vi "GV_AutoScale.vi"(8 "error in (no error)":errorcluster, 9 "AutoScale":T1, 11 "Gviewer in":refnum<class "Gviewer.lvclass">) -> (0 "error out":errorcluster, 3 "Gviewer out":refnum<class "Gviewer.lvclass">)   [LabVIEW 2020, in "Sgraph_lib_V1.lvlib" / "Gviewer.lvclass"]
doc: "Andre Koelewijn, 16 aug 2021\nPerform Autoscale action\nFix 29 dec 2021: skip autoscale if no data is present."
uses:
  Gviewer.lvclass
  controls/AutoScale.ctl
  Gviewer.lvclass/Gviewer.ctl
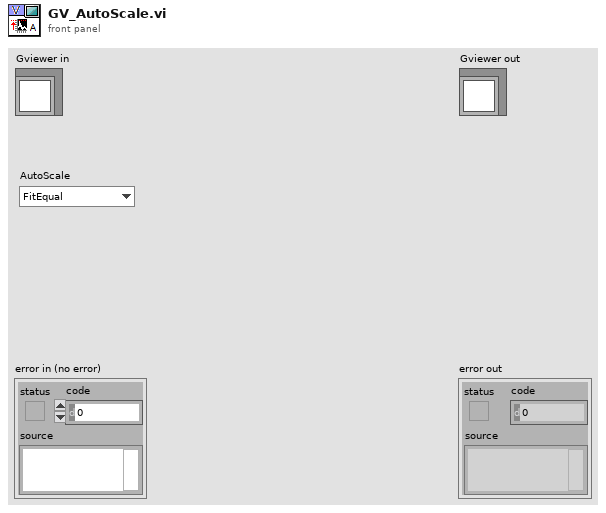
[diagram p1: front panel]
types:
  T1 = typedef "Sgraph_lib_V1.lvlib/Gviewer.lvclass/AutoScale.ctl" = enum16{"FitEqual", "FitMax", "StackEqual", "StackMax", "StackPerType"}
  T2 = typedef "Sgraph_lib_V1.lvlib/DBAL.lvclass/DBAL_TAGprops.ctl" = T3[]
  T3 = typedef "Sgraph_lib_V1.lvlib/DBAL.lvclass/DBAL_TAGpropEdit.ctl" = cluster{"TAG":string, "Qtype":string, "TAGprop":T4}
  T4 = typedef "Sgraph_lib_V1.lvlib/typedef_com_TagProp.ctl" = cluster{"Description":string, "EngUnits":string, "RangeH":dbl, "RangeL":dbl, "Resolution":i32, "Obsolete":bool, "ChangeDate":timestamp, "ChangeSource":string, "ChangeReason":string, "TagFunc":u32}
  T5 = cluster{"data":dbl[], "max":dbl[], "min":dbl[], "Status":u32[]}[]
  T6 = cluster{"data":dbl[], "max":dbl[], "min":dbl[], "Status":u32[]}
  T7 = typedef "Sgraph_lib_V1.lvlib/Gviewer.lvclass/Typedef_SelProperties.ctl" = cluster{"Color":u32, "LineType":T8, "max":dbl, "min":dbl}
  T8 = typedef "Sgraph_lib_V1.lvlib/Gviewer.lvclass/Typedef_LineType.ctl" = enum16{"num_bare", "num_MinMax_Area", "num_MinMax_Lines", "num_MinMax_Forfor", "num_Max_Area", "num_Max_Line", "num_Max_Forfor", "num_Min_Area", "num_Min_Line", "num_Min_Fosfor", "Boolean_Line_01", "Boolean_Area_01", "Boolean_Fosfor_01", "Boolean_Line_TF", "Boolean_Area_TF", "Boolean_Fosfor_TF", "Boolean_OnOff_Line", "Boolean_OnOff_Area", "Boolean_OnOff_Fosfor", "Boolean_spare", "StringEvent_Line", "StringEvent_TimeLine"}
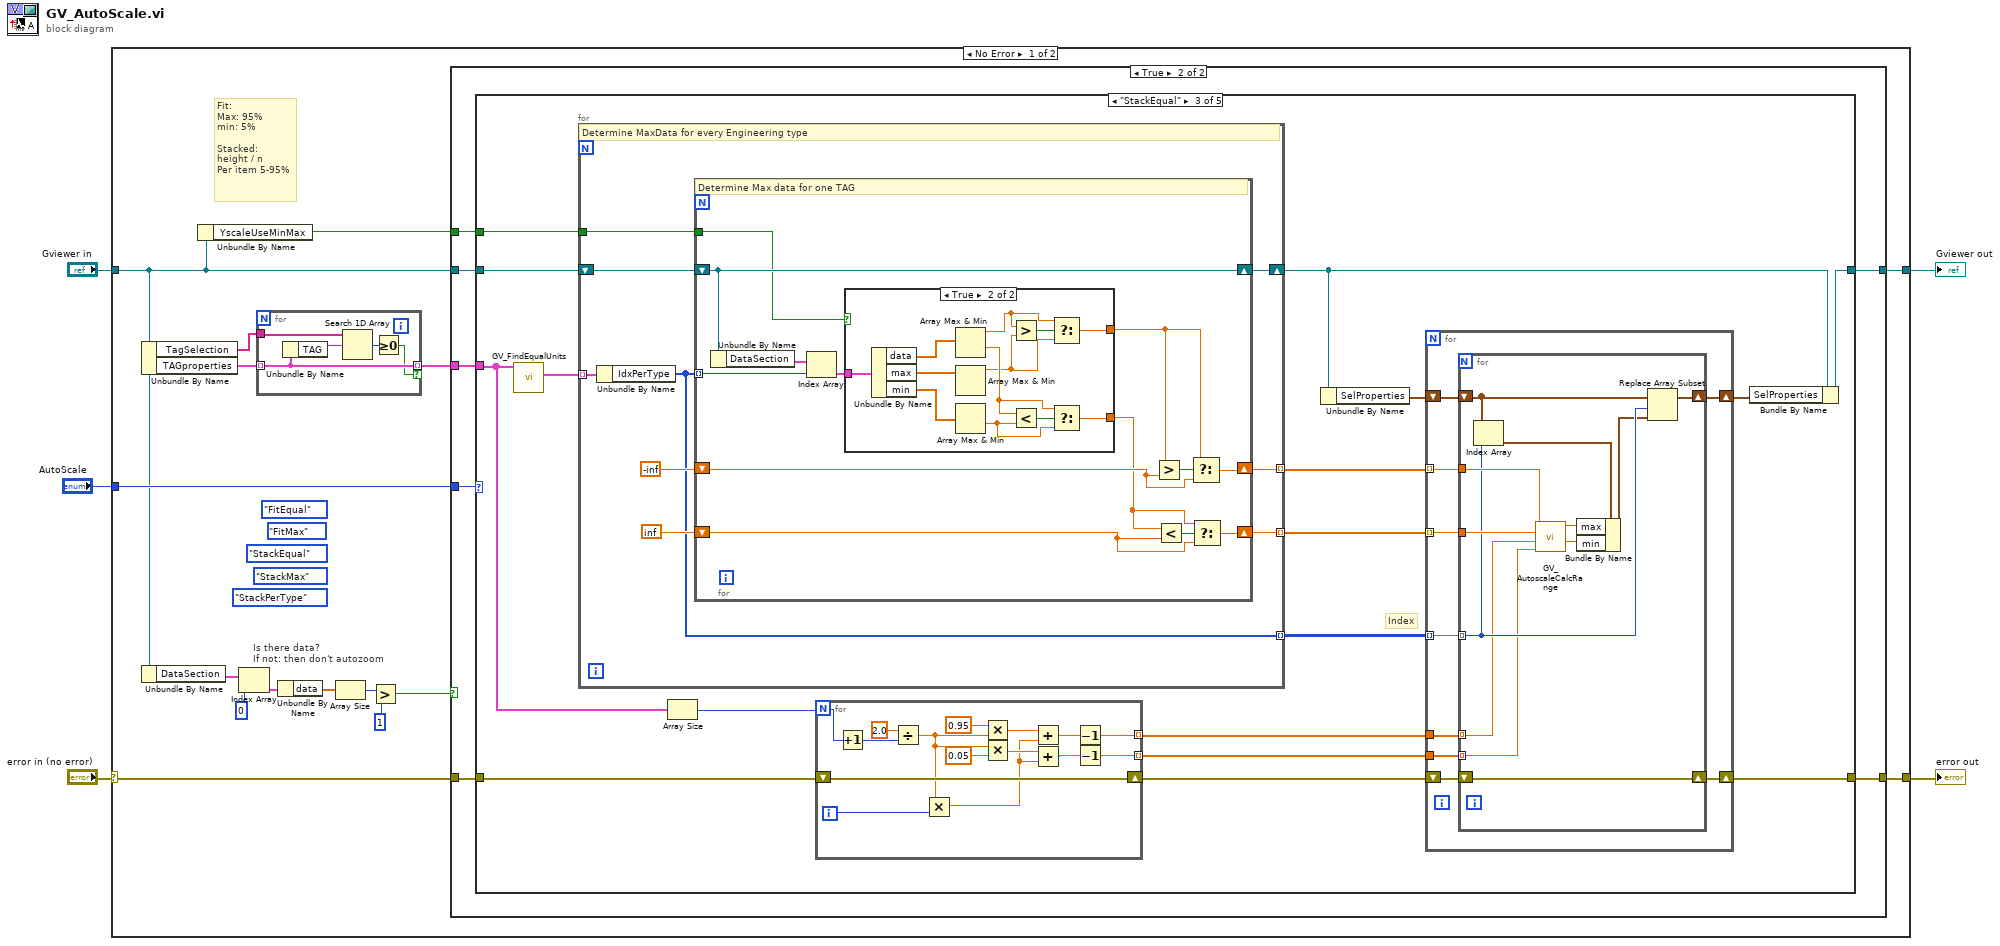
[diagram p0: block diagram]
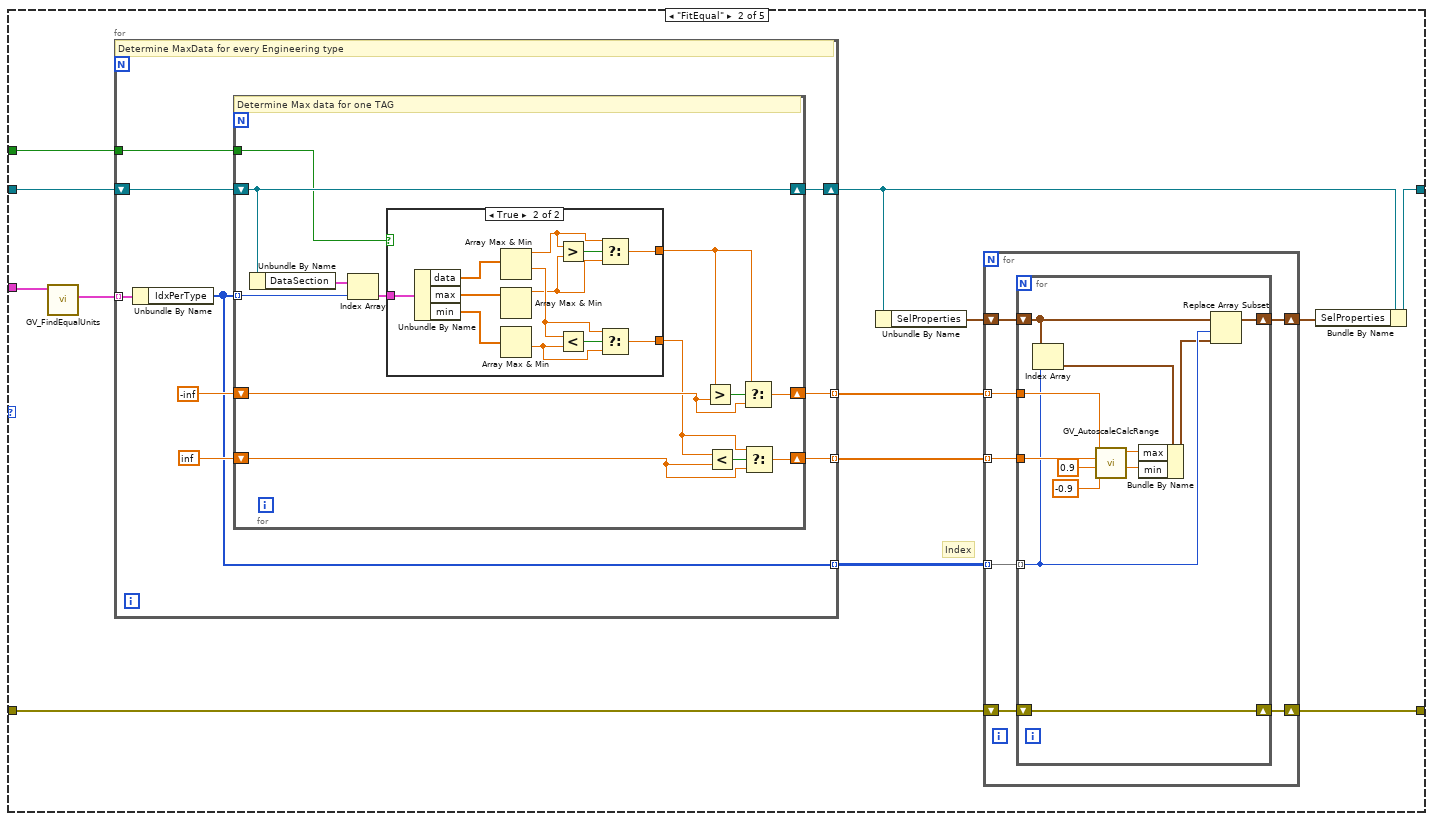
[diagram p4: hidden frame]
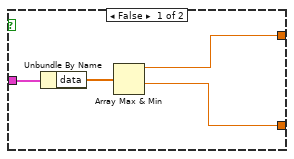
[diagram p5: hidden frame]
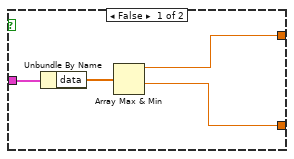
[diagram p6: hidden frame]
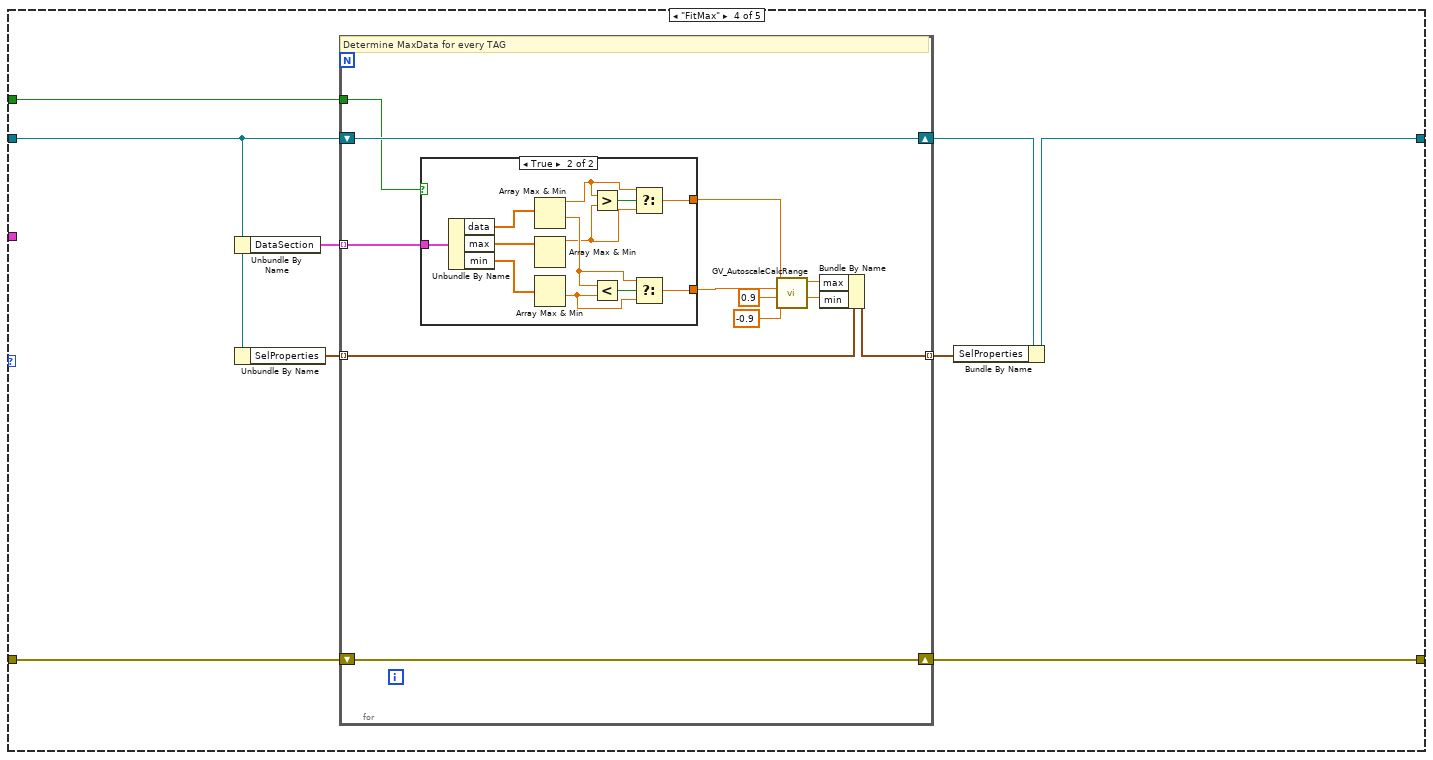
[diagram p7: hidden frame]
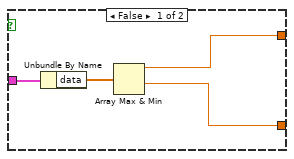
[diagram p8: hidden frame]
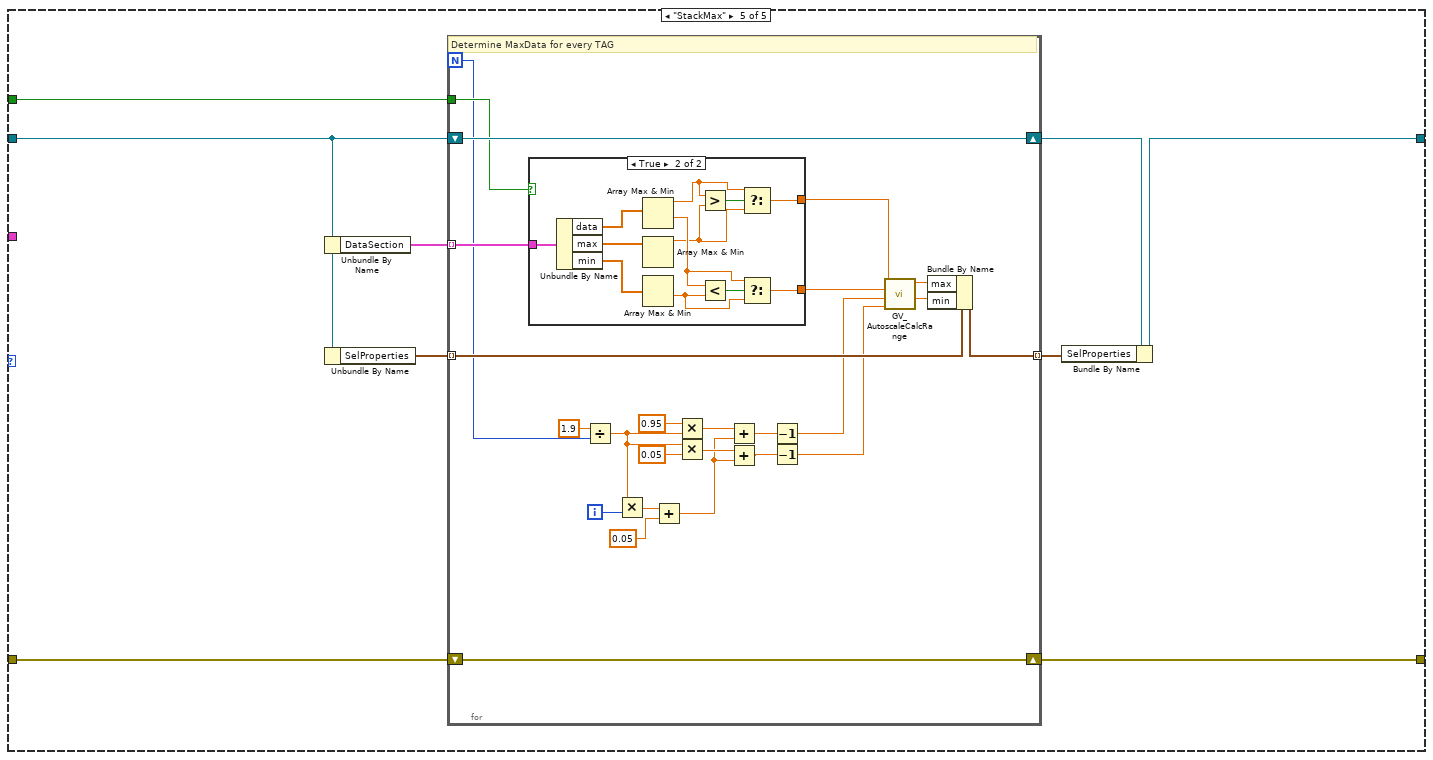
[diagram p9: hidden frame]
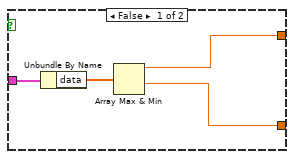
[diagram p10: hidden frame]
diagram:
  n1 = case shown="No Error" "error in (no error)" {
    selector: "error in (no error)" -> [w15 w284]
    tunnel: [w19 w284] -> w4
    tunnel: [w16 w283] -> w2
    tunnel: "Gviewer in" -> [w13 w283]
    tunnel: "AutoScale" -> [w17 _]
    frame No Error {
      (unwired) AutoScale."StackPerType" ("AutoScale")
      (unwired) AutoScale."StackMax" ("AutoScale")
      (unwired) AutoScale."StackEqual" ("AutoScale")
      (unwired) AutoScale."FitMax" ("AutoScale")
      (unwired) AutoScale."FitEqual" ("AutoScale")
      # "Is there data?\nIf not: then don't autozoom"
      # "Fit:\nMax: 95%\nmin: 5%\n\nStacked:\nheight / n\nPer item 5-95%"
      n2 = Unbundle By Name(w13) -> ("TagSelection"=w20:string[], "TAGproperties"=w21:T2)
      n3 = Unbundle By Name(w13) -> ("DataSection"=w12:T5)
      n4 = Unbundle By Name(w13) -> ("YscaleUseMinMax"=w14:bool)
      n5 = Index Array(array=w12, index=0) -> (element=w10:T6)
      n6 = for {
        tunnel: w21 -> [w282] mode=indexing
        tunnel: [w282] -> w18 mode=indexing if=w278
        tunnel: w20 -> [w281]
        n7 = Unbundle By Name(w282) -> ("TAG"=w280:string)
        n8 = Search 1D Array(1D array=w281, element=w280) -> (index of element=w279:i32)  [unwired: 1 in]
        n9 = Greater Or Equal To 0?(x=w279) -> (x >= 0?=w278:bool)
      }
      n10 = Unbundle By Name(w10) -> ("data"=w9:dbl[])
      n11 = Array Size(array=w9) -> (size(s)=w8:i32)
      n12 = Greater?(x=w8, y=1) -> (0:w6:bool)
      n13 = case shown="True" w6 {
        tunnel: [w22 w30] -> w19
        tunnel: w18 -> [_ w29]
        tunnel: w17 -> [_ w28]
        tunnel: [w23 w27] -> w16
        tunnel: w15 -> [w22 w26]
        tunnel: w14 -> [_ w25]
        tunnel: w13 -> [w23 w24]
        frame False {
        }
        frame True {
          n14 = case shown="\"StackEqual\"" w28 {
            tunnel: w26 -> [w32 w39 w104 w195 w234]
            tunnel: [w32 w39 w104 w191 w230] -> w30
            tunnel: w29 -> [_ w44 w106 _ _]
            tunnel: w24 -> [w31 w42 w115 w197 w228]
            tunnel: [w31 w33 w107 w192 w231] -> w27
            tunnel: w25 -> [_ w41 w114 w199 w236]
            frame Default {
            }
            frame "FitEqual" {
              # "Index"
              n15 = call "GV_FindEqualUnits.vi"("TAGproperties"=w44) -> ("IndexPerType"=w43:cluster{"EngUnit":string, "IdxPerType":i32[]}[])  [unwired: 8 in, 2 out]
              n16 = for {
                tunnel: w43 -> [w72] mode=indexing
                shift-right: [w71] -> w34
                shift-left: w42 -> [w70]
                tunnel: [w67] -> w38 mode=indexing
                tunnel: [w66] -> w37 mode=indexing
                tunnel: [w65] -> w40 mode=indexing
                tunnel: w41 -> [w64]
                # "Determine MaxData for every Engineering type"
                n17 = Unbundle By Name(w72) -> ("IdxPerType"=w65:i32[])
                n18 = for {
                  tunnel: w65 -> [w83] mode=indexing
                  shift-right: [w85] -> w71
                  shift-left: w70 -> [w85]
                  shift-right: [w79] -> w67
                  shift-left: -inf -> [w78]
                  shift-right: [w74] -> w66
                  shift-left: inf -> [w75]
                  tunnel: w64 -> [w73]
                  # "Determine Max data for one TAG"
                  n19 = Unbundle By Name(w85) -> ("DataSection"=w84:T5)
                  n20 = Index Array(array=w84, index=w83) -> (element=w82:T6)
                  n21 = case shown="True" w73 {
                    tunnel: w82 -> [w88 w101]
                    tunnel: [w87 w93] -> w80
                    tunnel: [w86 w92] -> w76
                    frame False {
                      n22 = Unbundle By Name(w88) -> ("data"=w89:dbl[])
                      n23 = Array Max & Min(array=w89) -> (max value=w87:dbl, min value=w86:dbl)  [unwired: 2 out]
                    }
                    frame True {
                      n24 = Unbundle By Name(w101) -> ("data"=w100:dbl[], "max"=w99:dbl[], "min"=w98:dbl[])
                      n25 = Array Max & Min(array=w100) -> (max value=w91:dbl, min value=w94:dbl)  [unwired: 2 out]
                      n26 = Array Max & Min(array=w99) -> (max value=w90:dbl)  [unwired: 3 out]
                      n27 = Array Max & Min(array=w98) -> (min value=w95:dbl)  [unwired: 3 out]
                      n28 = Greater?(x=w91, y=w90) -> (0:w97:bool)
                      n29 = Less?(x=w94, y=w95) -> (x < y?=w96:bool)
                      n30 = Select(t=w91, s=w97, f=w90) -> (s? t:f=w93:dbl)
                      n31 = Select(t=w94, s=w96, f=w95) -> (s? t:f=w92:dbl)
                    }
                  }
                  n32 = Greater?(x=w80, y=w78) -> (0:w81:bool)
                  n33 = Less?(x=w76, y=w75) -> (x < y?=w77:bool)
                  n34 = Select(t=w80, s=w81, f=w78) -> (s? t:f=w79:dbl)
                  n35 = Select(t=w76, s=w77, f=w75) -> (s? t:f=w74:dbl)
                }
              }
              n36 = Unbundle By Name(w34) -> ("SelProperties"=w36:T7[])
              n37 = for {
                tunnel: w40 -> [w51] mode=indexing
                shift-right: [w49] -> _
                shift-left: w39 -> [w50]
                tunnel: w38 -> [w48] mode=indexing
                tunnel: w37 -> [w47] mode=indexing
                shift-right: [w45] -> w35
                shift-left: w36 -> [w46]
                n38 = for {
                  tunnel: w51 -> [w56] mode=indexing
                  shift-right: [w63] -> w49
                  shift-left: w50 -> [w63]
                  tunnel: w48 -> [w60]
                  tunnel: w47 -> [w59]
                  shift-right: [w58] -> w45
                  shift-left: w46 -> [w57]
                  n39 = Index Array(array=w57, index=w56) -> (element=w55:T7)
                  n40 = call "GV_AutoscaleCalcRange.vi"("BottomVal"=-0.9, "TopVal"=0.9, "Min_data"=w59, "Max_data"=w60) -> ("Min Setting"=w52:dbl, "Max Setting"=w53:dbl)  [unwired: 6 in]
                  n41 = Bundle By Name(cluster=w55, "max"=w53, "min"=w52) -> (w54:T7)
                  n42 = Replace Array Subset(array=w57, new element=w54, index=w56) -> (w58:T7[])
                }
              }
              n43 = Bundle By Name(cluster=w34, "SelProperties"=w35) -> (w33:refnum<class "Gviewer.lvclass">)
            }
            frame "StackEqual" {
              # "Index"
              n44 = call "GV_FindEqualUnits.vi"("TAGproperties"=w106) -> ("IndexPerType"=w116:cluster{"EngUnit":string, "IdxPerType":i32[]}[])  [unwired: 8 in, 2 out]
              n45 = for {
                tunnel: w116 -> [w161] mode=indexing
                shift-right: [w160] -> w108
                shift-left: w115 -> [w159]
                tunnel: [w156] -> w112 mode=indexing
                tunnel: [w155] -> w111 mode=indexing
                tunnel: [w154] -> w113 mode=indexing
                tunnel: w114 -> [w153]
                # "Determine MaxData for every Engineering type"
                n46 = Unbundle By Name(w161) -> ("IdxPerType"=w154:i32[])
                n47 = for {
                  tunnel: w154 -> [w172] mode=indexing
                  shift-right: [w174] -> w160
                  shift-left: w159 -> [w174]
                  shift-right: [w168] -> w156
                  shift-left: -inf -> [w167]
                  shift-right: [w163] -> w155
                  shift-left: inf -> [w164]
                  tunnel: w153 -> [w162]
                  # "Determine Max data for one TAG"
                  n48 = Unbundle By Name(w174) -> ("DataSection"=w173:T5)
                  n49 = Index Array(array=w173, index=w172) -> (element=w171:T6)
                  n50 = case shown="True" w162 {
                    tunnel: w171 -> [w177 w190]
                    tunnel: [w176 w182] -> w169
                    tunnel: [w175 w181] -> w165
                    frame False {
                      n51 = Unbundle By Name(w177) -> ("data"=w178:dbl[])
                      n52 = Array Max & Min(array=w178) -> (max value=w176:dbl, min value=w175:dbl)  [unwired: 2 out]
                    }
                    frame True {
                      n53 = Unbundle By Name(w190) -> ("data"=w189:dbl[], "max"=w188:dbl[], "min"=w187:dbl[])
                      n54 = Array Max & Min(array=w189) -> (max value=w180:dbl, min value=w183:dbl)  [unwired: 2 out]
                      n55 = Array Max & Min(array=w188) -> (max value=w179:dbl)  [unwired: 3 out]
                      n56 = Array Max & Min(array=w187) -> (min value=w184:dbl)  [unwired: 3 out]
                      n57 = Greater?(x=w180, y=w179) -> (0:w186:bool)
                      n58 = Less?(x=w183, y=w184) -> (x < y?=w185:bool)
                      n59 = Select(t=w180, s=w186, f=w179) -> (s? t:f=w182:dbl)
                      n60 = Select(t=w183, s=w185, f=w184) -> (s? t:f=w181:dbl)
                    }
                  }
                  n61 = Greater?(x=w169, y=w167) -> (0:w170:bool)
                  n62 = Less?(x=w165, y=w164) -> (x < y?=w166:bool)
                  n63 = Select(t=w169, s=w170, f=w167) -> (s? t:f=w168:dbl)
                  n64 = Select(t=w165, s=w166, f=w164) -> (s? t:f=w163:dbl)
                }
              }
              n65 = Array Size(array=w106) -> (size(s)=w105:i32)
              n66 = for {
                N: w105 -> [w129]
                shift-right: [w131] -> _
                shift-left: w104 -> [w131]
                tunnel: [w118] -> w103 mode=indexing
                tunnel: [w117] -> w102 mode=indexing
                i -> [w127]
                n67 = Increment(x=w129) -> (x+1=w128:i32)
                n68 = Divide(x=2.0, y=w128) -> (x/y=w125:dbl)
                n69 = Multiply(x=w125, y=w127) -> (x*y=w121:dbl)
                n70 = Multiply(x=0.95, y=w125) -> (x*y=w123:dbl)
                n71 = Multiply(x=w125, y=0.05) -> (x*y=w122:dbl)
                n72 = Add(x=w123, y=w121) -> (x+y=w120:dbl)
                n73 = Add(x=w122, y=w121) -> (x+y=w119:dbl)
                n74 = Decrement(x=w120) -> (x-1=w118:dbl)
                n75 = Decrement(x=w119) -> (x-1=w117:dbl)
              }
              n76 = Unbundle By Name(w108) -> ("SelProperties"=w110:T7[])
              n77 = for {
                tunnel: w113 -> [w140] mode=indexing
                shift-right: [w138] -> _
                shift-left: w104 -> [w139]
                tunnel: w112 -> [w137] mode=indexing
                tunnel: w111 -> [w136] mode=indexing
                shift-right: [w134] -> w109
                shift-left: w110 -> [w135]
                tunnel: w103 -> [w133]
                tunnel: w102 -> [w132]
                n78 = for {
                  tunnel: w140 -> [w147] mode=indexing
                  shift-right: [w152] -> w138
                  shift-left: w139 -> [w152]
                  tunnel: w137 -> [w151]
                  tunnel: w136 -> [w150]
                  shift-right: [w149] -> w134
                  shift-left: w135 -> [w148]
                  tunnel: w133 -> [w142] mode=indexing
                  tunnel: w132 -> [w141] mode=indexing
                  n79 = Index Array(array=w148, index=w147) -> (element=w146:T7)
                  n80 = call "GV_AutoscaleCalcRange.vi"("BottomVal"=w141, "TopVal"=w142, "Min_data"=w150, "Max_data"=w151) -> ("Min Setting"=w143:dbl, "Max Setting"=w144:dbl)  [unwired: 6 in]
                  n81 = Bundle By Name(cluster=w146, "max"=w144, "min"=w143) -> (w145:T7)
                  n82 = Replace Array Subset(array=w148, new element=w145, index=w147) -> (w149:T7[])
                }
              }
              n83 = Bundle By Name(cluster=w108, "SelProperties"=w109) -> (w107:refnum<class "Gviewer.lvclass">)
            }
            frame "FitMax" {
              n84 = Unbundle By Name(w197) -> ("DataSection"=w198:T5)
              n85 = Unbundle By Name(w197) -> ("SelProperties"=w196:T7[])
              n86 = for {
                shift-right: [w211] -> w193
                shift-left: w197 -> [w211]
                tunnel: w199 -> [w210]
                tunnel: w198 -> [w209] mode=indexing
                tunnel: w196 -> [w204] mode=indexing
                tunnel: [w203] -> w194 mode=indexing
                shift-right: [w200] -> w191
                shift-left: w195 -> [w200]
                # "Determine MaxData for every TAG"
                n87 = case shown="True" w210 {
                  tunnel: w209 -> [w214 w227]
                  tunnel: [w213 w219] -> w202
                  tunnel: [w212 w218] -> w201
                  frame False {
                    n88 = Unbundle By Name(w214) -> ("data"=w215:dbl[])
                    n89 = Array Max & Min(array=w215) -> (max value=w213:dbl, min value=w212:dbl)  [unwired: 2 out]
                  }
                  frame True {
                    n90 = Unbundle By Name(w227) -> ("data"=w226:dbl[], "max"=w225:dbl[], "min"=w224:dbl[])
                    n91 = Array Max & Min(array=w226) -> (max value=w217:dbl, min value=w220:dbl)  [unwired: 2 out]
                    n92 = Array Max & Min(array=w225) -> (max value=w216:dbl)  [unwired: 3 out]
                    n93 = Array Max & Min(array=w224) -> (min value=w221:dbl)  [unwired: 3 out]
                    n94 = Greater?(x=w217, y=w216) -> (0:w223:bool)
                    n95 = Less?(x=w220, y=w221) -> (x < y?=w222:bool)
                    n96 = Select(t=w217, s=w223, f=w216) -> (s? t:f=w219:dbl)
                    n97 = Select(t=w220, s=w222, f=w221) -> (s? t:f=w218:dbl)
                  }
                }
                n98 = call "GV_AutoscaleCalcRange.vi"("BottomVal"=-0.9, "TopVal"=0.9, "Min_data"=w201, "Max_data"=w202) -> ("Min Setting"=w208:dbl, "Max Setting"=w207:dbl)  [unwired: 6 in]
                n99 = Bundle By Name(cluster=w204, "max"=w207, "min"=w208) -> (w203:T7)
              }
              n100 = Bundle By Name(cluster=w193, "SelProperties"=w194) -> (w192:refnum<class "Gviewer.lvclass">)
            }
            frame "StackMax" {
              n101 = Unbundle By Name(w228) -> ("DataSection"=w229:T5)
              n102 = Unbundle By Name(w228) -> ("SelProperties"=w235:T7[])
              n103 = for {
                N -> [w240]
                shift-right: [w261] -> w232
                shift-left: w228 -> [w261]
                tunnel: w236 -> [w260]
                tunnel: w229 -> [w259] mode=indexing
                tunnel: w235 -> [w256] mode=indexing
                tunnel: [w255] -> w233 mode=indexing
                shift-right: [w252] -> w230
                shift-left: w234 -> [w252]
                i -> [w243]
                # "Determine MaxData for every TAG"
                n104 = case shown="True" w260 {
                  tunnel: w259 -> [w264 w277]
                  tunnel: [w263 w269] -> w254
                  tunnel: [w262 w268] -> w253
                  frame False {
                    n105 = Unbundle By Name(w264) -> ("data"=w265:dbl[])
                    n106 = Array Max & Min(array=w265) -> (max value=w263:dbl, min value=w262:dbl)  [unwired: 2 out]
                  }
                  frame True {
                    n107 = Unbundle By Name(w277) -> ("data"=w276:dbl[], "max"=w275:dbl[], "min"=w274:dbl[])
                    n108 = Array Max & Min(array=w276) -> (max value=w267:dbl, min value=w270:dbl)  [unwired: 2 out]
                    n109 = Array Max & Min(array=w275) -> (max value=w266:dbl)  [unwired: 3 out]
                    n110 = Array Max & Min(array=w274) -> (min value=w271:dbl)  [unwired: 3 out]
                    n111 = Greater?(x=w267, y=w266) -> (0:w273:bool)
                    n112 = Less?(x=w270, y=w271) -> (x < y?=w272:bool)
                    n113 = Select(t=w267, s=w273, f=w266) -> (s? t:f=w269:dbl)
                    n114 = Select(t=w270, s=w272, f=w271) -> (s? t:f=w268:dbl)
                  }
                }
                n115 = Divide(x=1.9, y=w240) -> (x/y=w249:dbl)
                n116 = Multiply(x=w249, y=w243) -> (x*y=w239:dbl)
                n117 = Add(x=w239, y=0.05) -> (x+y=w237:dbl)
                n118 = Multiply(x=0.95, y=w249) -> (x*y=w247:dbl)
                n119 = Multiply(x=w249, y=0.05) -> (x*y=w246:dbl)
                n120 = Add(x=w247, y=w237) -> (x+y=w245:dbl)
                n121 = Add(x=w246, y=w237) -> (x+y=w244:dbl)
                n122 = Decrement(x=w245) -> (x-1=w242:dbl)
                n123 = Decrement(x=w244) -> (x-1=w241:dbl)
                n124 = call "GV_AutoscaleCalcRange.vi"("BottomVal"=w241, "TopVal"=w242, "Min_data"=w253, "Max_data"=w254) -> ("Min Setting"=w258:dbl, "Max Setting"=w257:dbl)  [unwired: 6 in]
                n125 = Bundle By Name(cluster=w256, "max"=w257, "min"=w258) -> (w255:T7)
              }
              n126 = Bundle By Name(cluster=w232, "SelProperties"=w233) -> (w231:refnum<class "Gviewer.lvclass">)
            }
          }
        }
      }
    }
    frame Error {
    }
  }
  "error out" <- w4
  "Gviewer out" <- w2
